vi "TDMS Advanced Overwrite.vi"   [LabVIEW 2023]
doc: "This example demonstrates how to overwrite data from a specified position by using the Advanced TDMS VIs and functions."
uses:
  <vilib>/Utility/TDMS File Viewer/NI_TDMS File Viewer.lvlib
panel:
  # "Overview: Demonstrates the use of the Advanced TDMS functions to overwrite a .tdms file.\nInstructions:\n1. Make sure you have already run TDMS Advanced Asynchronous Write.vi.\n2. Run this VI.\n3. Delete the TDMS file (located at [LabVIEW Data]\\Example TDMS Advanced Asynchronous Write.tdms) when you are done."
types:
  T1 = enum16{"open", "open or create", "create or replace", "create", "open (read-only)"}
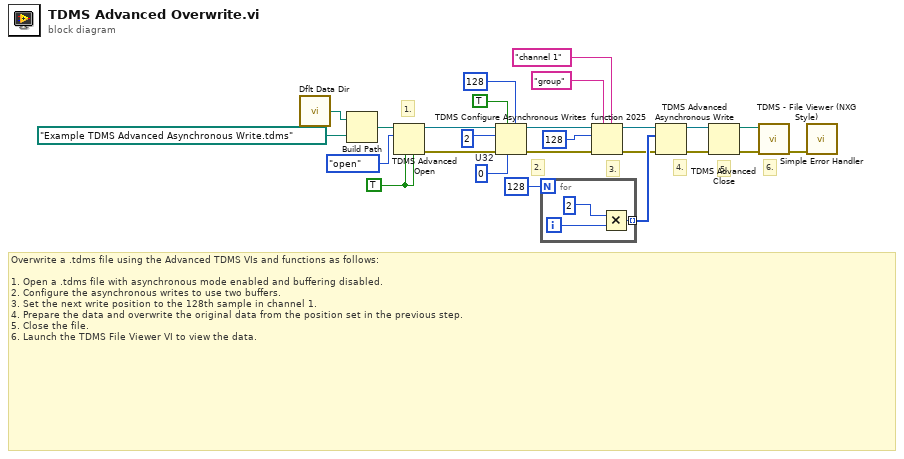
[diagram p0: block diagram]
diagram:
  w19 = u32 0  # U32
  w21 = TRUE ("enable asynchronous? (T)")
  # "6."
  # "4."
  # "3."
  # "2."
  # "Overwrite a .tdms file using the Advanced TDMS VIs and functions as follows:\n\n1. Open a .tdms file with asynchronous mode enabled and buffering disabled.\n2. Configure the asynchronous writes to use two buffers.\n3. Set the next write position to the 128th sample in channel 1.\n4. Prepare the data and overwrite the original data from the position set in the previous step.\n5. Close the file.\n6. Launch the TDMS File Viewer VI to view the data."
  # "1."
  # "5."
  n1 = call <vilib>:"Dflt Data Dir.vi"() -> ("App:Default Data Directory"=w22:path)
  n2 = Build Path(base path=w22, name or relative path=path "Example TDMS Advanced Asynchronous Write.tdms") -> (appended path=w24:path)
  n3 = TDMS Advanced Open(4:w21, 6:w21, 10:T1."open" ("operation (0:open)"), 11:w24) -> (0:w12:errorcluster, 3:w11:refnum<k34>)  [unwired: 1 in, 1 out]
  n4 = TDMS Configure Asynchronous Writes(5:u32 128 ("max write size"), 6:w19, 7:TRUE ("pre-allocate? (F)"), 8:w12, 10:u32 2 ("max asynchronous writes (4)"), 11:w11) -> (0:w9:errorcluster, 3:w10:refnum<k34>)  [unwired: 1 in]
  n5 = for {
    N: 128 -> [_]
    tunnel: [w27] -> w13 mode=indexing
    i -> [w28]
    n6 = Multiply(x=2, y=w28) -> (x*y=w27:i32)
  }
  n7 = fn#2025(5:"channel 1" ("channel name in"), 7:"group" ("group name in"), 8:w9, 10:i64 128 ("offset (0)"), 11:w10) -> (0:w6:errorcluster, 3:w8:refnum<k34>)  [unwired: 1 in]
  n8 = TDMS Advanced Asynchronous Write(8:w6, 10:w13, 11:w8) -> (0:w5:errorcluster, 3:w7:refnum<k34>)
  n9 = TDMS Advanced Close(8:w5, 11:w7) -> (0:w4:errorcluster, 3:w2:path)  [unwired: 2 in]
  n10 = call <vilib>:"TDMS - File Viewer (NXG Style).vi"("error in"=w4, "file in"=w2) -> ("error out"=w3:errorcluster)  [unwired: 8 in, 1 out]
  n11 = call <vilib>:"Simple Error Handler.vi"("error in (no error)"=w3) -> ()  [unwired: 4 in, 5 out]
